vi "StatusOnlyResult.vi"(8 "error in (no error)":errorcluster, 11 "map":map{string, string}(c390)) -> (0 "error out":errorcluster, 2 "status":string)   [LabVIEW 2021]
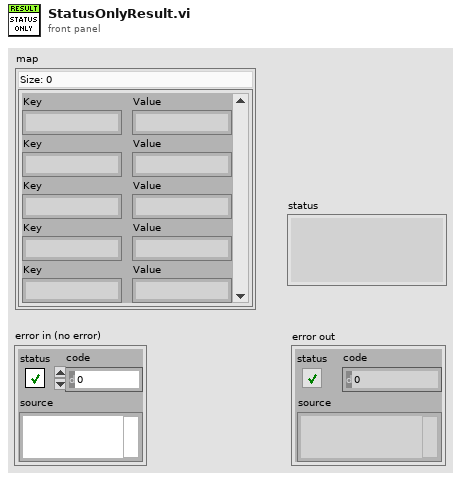
[diagram p1: front panel]
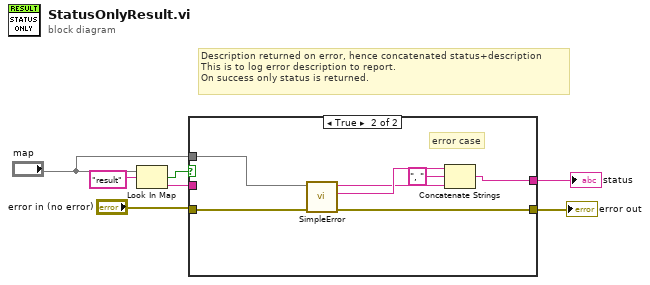
[diagram p0: block diagram]
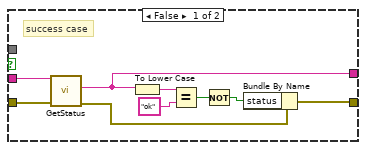
[diagram p2: hidden frame]
diagram:
  # "Description returned on error, hence concatenated status+description\nThis is to log error description to report.\nOn success only status is returned."
  n1 = Look In Map(map="map", key="result") -> (key not found?=w5:bool, value=w6:string)  [unwired: 1 in]
  n2 = case shown="True" w5 {
    tunnel: w6 -> [w15 _]
    tunnel: "error in (no error)" -> [w16 w23]
    tunnel: [w9 w22] -> w3
    tunnel: "map" -> [_ w21]
    tunnel: [w8 w17] -> w1
    frame False {
      # "success case"
      n3 = call "GetStatus.vi"("error in (no error)"=w16, "Value"=w15) -> ("error out"=w10:errorcluster, "status"=w8:string)  [unwired: 7 in, 1 out]
      n4 = To Lower Case(string=w8) -> (all lower case string=w11:string)
      n5 = Equal?(x=w11, y="ok" ("regular expression")) -> (x = y?=w13:bool)
      n6 = Not(x=w13) -> (.not. x?=w12:bool)
      n7 = Bundle By Name(cluster=w10, "status"=w12) -> (w9:errorcluster)
    }
    frame True {
      # "error case"
      n8 = call "SimpleError.vi"("error in (no error)"=w23, "map"=w21) -> ("error out"=w22:errorcluster, "status"=w20:string, "description"=w18:string)  [unwired: 7 in]
      n9 = Concatenate Strings(w20, ", " ("string"), w18) -> (w17:string)
    }
  }
  "error out" <- w3
  "status" <- w1
